vi "TestExe Path.vi"() -> (1 "Application : nom":string, 2 "En Exe?":bool, 3 "Chemin Actuel":path)   [LabVIEW 2020, in "Library Commun.lvlib"]
uses:
  Commun VI/Library Commun.lvlib
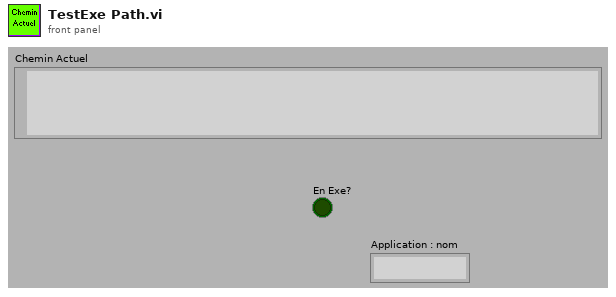
[diagram p1: front panel]
types:
  T1 = enum32{"invalid app kind", "Development System", "Run Time System", "Student Edition", "Embedded LabVIEW", "Evaluation", "Custom"}
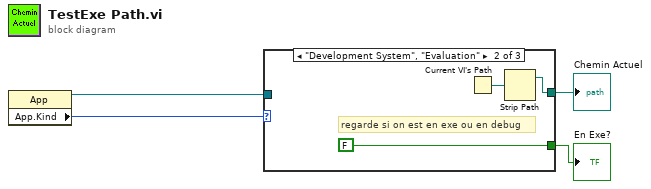
[diagram p0: block diagram]
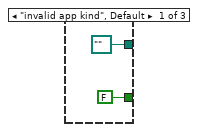
[diagram p2: hidden frame]
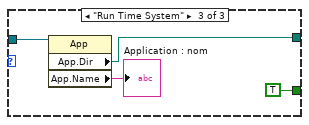
[diagram p3: hidden frame]
diagram:
  n1 = property class="App"() -> (reference out=w2:refnum<vi>, "App.Kind"=w4:T1)  [unwired: 2 in, 1 out]
  n2 = case shown="\"Development System\", \"Evaluation\"" w4 {
    tunnel: [FALSE FALSE TRUE] -> w3
    tunnel: [path "" ("App.Dir") w7 w11] -> w1
    tunnel: w2 -> [_ _ w12]
    frame "invalid app kind", Default {
    }
    frame "Development System", "Evaluation" {
      # "regarde si on est en exe ou en debug"
      n3 = Current VI's Path() -> (path=w8:path)
      n4 = Strip Path(path=w8) -> (stripped path=w7:path)  [unwired: 1 out]
    }
    frame "Run Time System" {
      n5 = property class="App"(reference=w12) -> ("App.Dir"=w11:path, "App.Name"=→"Application : nom":string)  [unwired: 1 in, 2 out]
    }
  }
  "En Exe?" <- w3
  "Chemin Actuel" <- w1
